vi "Throw Error if Invalid Path.vi"(8 "error in":errorcluster, 9 "is archive path":bool, 10 "file path":path, 11 "item reference in":T1 format="%.0x") -> (0 "error out":errorcluster, 3 "item reference out":T1 format="%.0x")   [LabVIEW 2027, in "Embedded Data Logger System Explorer.lvlib"]
uses:
  Embedded Data Logger System Explorer.lvlib
  <vilib>/NI VeriStand/Custom Device API/Custom Device Item Ref.ctl
  <vilib>/NI VeriStand/Custom Device API/Custom Device API.lvlib
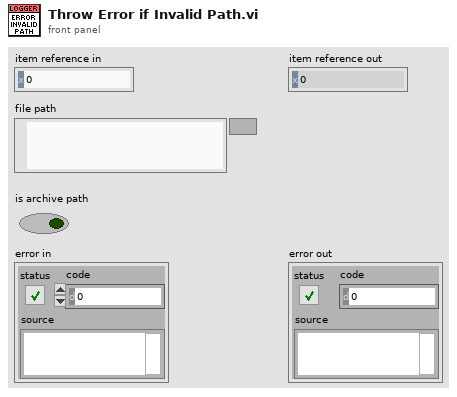
[diagram p1: front panel]
types:
  T1 = typedef "Custom Device API.lvlib/Custom Device Item Ref.ctl" = u64
  T2 = typedef "Custom Device API.lvlib/Custom Device Target Type.ctl" = enum16{"PharLap", "VxWorks", "Windows", "Linux_32_ARM", "Linux_x64"}
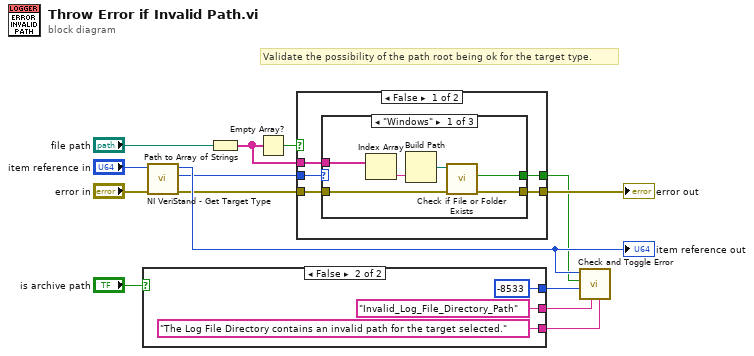
[diagram p0: block diagram]
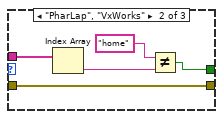
[diagram p2: hidden frame]
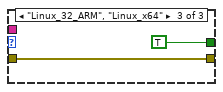
[diagram p3: hidden frame]
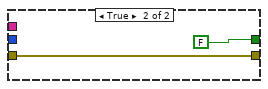
[diagram p4: hidden frame]
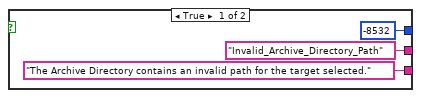
[diagram p5: hidden frame]
diagram:
  # "Validate the possibility of the path root being ok for the target type."
  n1 = case shown="False" "is archive path" {
    tunnel: [-8532 ("Error Code") -8533 ("Error Code")] -> w14
    tunnel: ["Invalid_Archive_Directory_Path" ("Error Key") "Invalid_Log_File_Directory_Path" ("Error Key")] -> w13
    tunnel: ["The Archive Directory contains an invalid path for the target selected." ("Error String") "The Log File Directory contains an invalid path for the target selected." ("Error String")] -> w12
    frame True {
    }
    frame False {
    }
  }
  n2 = call <vilib>:"NI VeriStand - Get Target Type.vi"("error in (no error)"="error in", "Item Ref in"="item reference in") -> ("error out"=w2:errorcluster, "Target Type"=w1:T2, "Item Ref out"=w9:T1)  [unwired: 7 in]
  "item reference out" <- w9
  n3 = Path to Array of Strings(0:"file path") -> (2:w7:string[])  [unwired: 1 out]
  n4 = Empty Array?(array=w7) -> (empty?=w6:bool)
  n5 = case shown="False" w6 {
    tunnel: w1 -> [w25 _]
    tunnel: [w24 FALSE ("file or folder exists?")] -> w4
    tunnel: w2 -> [w23 w40]
    tunnel: [w22 w40] -> w5
    tunnel: w7 -> [w21 _]
    frame False {
      n6 = case shown="\"Windows\"" w25 {
        tunnel: w21 -> [w31 w36 _]
        tunnel: [w29 w32 TRUE ("file or folder exists?")] -> w24
        tunnel: w23 -> [w28 w35 w37]
        tunnel: [w27 w35 w37] -> w22
        frame "Windows" {
          n7 = Index Array(array=w31) -> (element=w30:string)  [unwired: 1 in]
          n8 = Build Path(name or relative path=w30) -> (appended path=w26:path)  [unwired: 1 in]
          n9 = call <vilib>:"Check if File or Folder Exists.vi"("error in (no error)"=w28, "path"=w26) -> ("error out"=w27:errorcluster, "file or folder exists?"=w29:bool)  [unwired: 7 in, 1 out]
        }
        frame "PharLap", "VxWorks" {
          n10 = Index Array(array=w36) -> (element=w34:string)  [unwired: 1 in]
          n11 = Not Equal?(x="home", y=w34) -> (x != y?=w32:bool)
        }
        frame "Linux_32_ARM", "Linux_x64" {
        }
      }
    }
    frame True {
    }
  }
  "error out" <- w5
  n12 = call "Check and Toggle Error.vi"("error string"=w12, "error key"=w13, "error code"=w14, "clear error"=w4, "item reference in"=w9) -> ()  [unwired: 5 in, 2 out]
